vi "testReentrancy -- Easy Parse XML.vi"(8 "error in (no error)":errorcluster, 11 "TestCase in":refnum<class "EasyXMLTest.lvclass">) -> (0 "error out":errorcluster, 3 "TestCase out":refnum<class "EasyXMLTest.lvclass">)   [LabVIEW 2013, in "EasyXMLTest.lvclass"]
doc: "Verify that error in is not overwritten"
uses:
  EasyXMLTest.lvclass
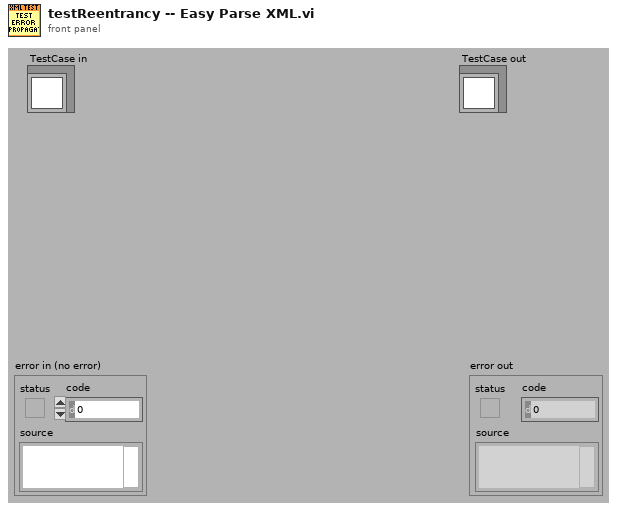
[diagram p1: front panel]
types:
  T1 = enum16{"Share clones between instances", "Preallocate clone for each instance"}
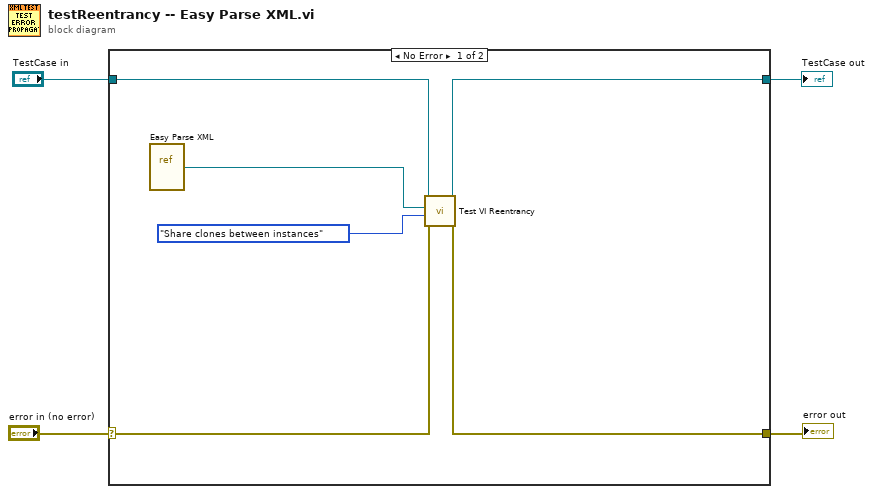
[diagram p0: block diagram]
diagram:
  n1 = case shown="No Error" "error in (no error)" {
    selector: "error in (no error)" -> [w8 w12]
    tunnel: [w9 w12] -> w3
    tunnel: [w10 w11] -> w1
    tunnel: "TestCase in" -> [w7 w11]
    frame No Error {
      n2 = vi-ref "Easy Parse XML.vi"() -> (w6:refnum<vi>)
      n3 = call "Test VI Reentrancy.vi"("error in (no error)"=w8, "Execution:Reentrancy Type"=T1."Share clones between instances", "VI Refnum"=w6, "TestCase in"=w7) -> ("error out"=w9:errorcluster, "TestCase out"=w10:refnum<class "EasyXMLTest.lvclass">)  [unwired: 6 in]
    }
    frame Error {
    }
  }
  "error out" <- w3
  "TestCase out" <- w1
